vi "Compute Calibration Phasor & jw.vi"(6 "Gate Width":dbl[unit], 7 "Harmonic frequency":dbl[unit], 8 "Laser Period":dbl[unit], 9 "# Gates":dbl, 10 "Calibration Lifetime":dbl[unit], 11 "Calibration Phasor Type":T1) -> (1 "z (tau_cal)":cdb, 3 "i 2 pi f (GHz)":cdb)   [LabVIEW 2019]
doc: "z (tau_cal) is the phasor calculated for tau_cal in either the UC_00 case (standard universal semicircle) or the UC_N case (discrete phasor of ungated periodic single-exponential decay), depending on the selected Calibration Phasor Type"
uses:
  Phasor Type.ctl
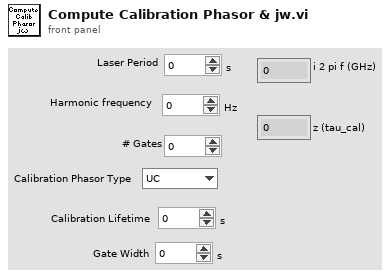
[diagram p1: front panel]
types:
  T1 = typedef "Phasor Type.ctl" = enum16{"UC", "L_N", "L_N[W]"}
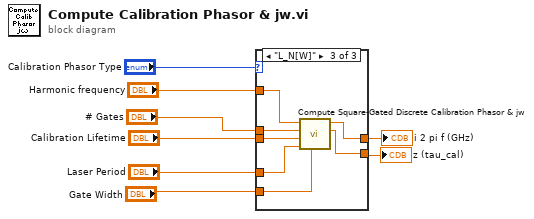
[diagram p0: block diagram]
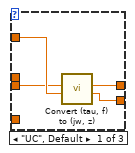
[diagram p2: hidden frame]
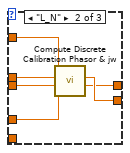
[diagram p3: hidden frame]
diagram:
  n1 = case shown="\"L_N[W]\"" "Calibration Phasor Type" {
    tunnel: "Harmonic frequency" -> [w12 w18 w25]
    tunnel: [w11 w13 w21] -> w3
    tunnel: [w10 w14 w20] -> w4
    tunnel: "Calibration Lifetime" -> [w9 w16 w23]
    tunnel: "# Gates" -> [_ w17 w24]
    tunnel: "Laser Period" -> [_ w15 w22]
    tunnel: "Gate Width" -> [_ _ w19]
    frame "UC", Default {
      n2 = call "Convert (tau, f) to (jw, z).vi"("Harmonic Frequency"=w12, "Lifetime"=w9) -> ("Phasor"=w10:cdb, "i 2 pi f (GHz)"=w11:cdb)  [unwired: 8 in]
    }
    frame "L_N" {
      n3 = call "Compute Discrete Calibration Phasor & jw.vi"("Laser Period (T)"=w15, "Calibration Lifetime (tau)"=w16, "# Gates (N)"=w17, "Harmonic frequency (f)"=w18) -> ("Z_N(tau)"=w14:cdb, "i 2 pi f (GHz)"=w13:cdb)  [unwired: 6 in]
    }
    frame "L_N[W]" {
      n4 = call "Compute Square-Gated Discrete Calibration Phasor & jw.vi"("Gate Width (W)"=w19, "Laser Period (T)"=w22, "Calibration Lifetime (tau)"=w23, "# Gates (N)"=w24, "Harmonic frequency (f)"=w25) -> ("Z_N[W](tau)/Z_N[W](0)"=w20:cdb, "i 2 pi f (GHz)"=w21:cdb)  [unwired: 5 in]
    }
  }
  "z (tau_cal)" <- w4
  "i 2 pi f (GHz)" <- w3
